vi "Retrieve Async Section configuration properties (interactions).vi"(8 "error in":errorcluster, 11 "section item ref in":T2 format="%.0x") -> (0 "error out":errorcluster, 1 "status channel configuration":map{string, map{string, i32}}(c390), 2 "data channel configuration":T1[](array[typedef]), 3 "section item ref out":T2 format="%.0x", 4 "Found":bool)   [LabVIEW 2019, in "HLA Custom Device System Explorer.lvlib"]
uses:
  HLA Custom Device System Explorer.lvlib
  <vilib>/NI VeriStand/Custom Device API/Custom Device Item Ref.ctl
  Shared/interaction_parameter_configuration.ctl
  Shared/Constants.vi
  <vilib>/NI VeriStand/Custom Device API/Get Item Property (String).vi
  <vilib>/NI VeriStand/Custom Device API/Custom Device API.lvlib
  Shared/HLA Custom Device Shared.lvlib
  <vilib>/NI VeriStand/Custom Device Tools/Custom Device Utility Library/Custom Device Utility Library.lvlib
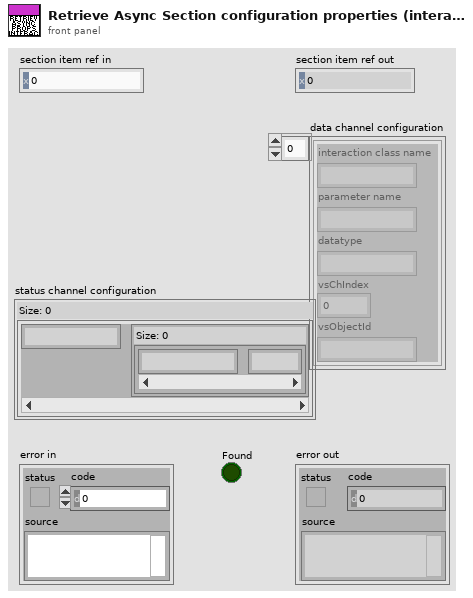
[diagram p1: front panel]
types:
  T1 = typedef "HLA Custom Device Shared.lvlib/interaction_parameter_configuration.ctl" = cluster{"interaction class name":string, "parameter name":string, "datatype":string, "vsChIndex":i32, "vsObjectId":string}
  T2 = typedef "Custom Device API.lvlib/Custom Device Item Ref.ctl" = u64
  T3 = typedef "Custom Device API.lvlib/Custom Device Item Info.ctl" = cluster{"Name":string, "Is Channel":bool, "GUID":string, "Is Waveform":bool}
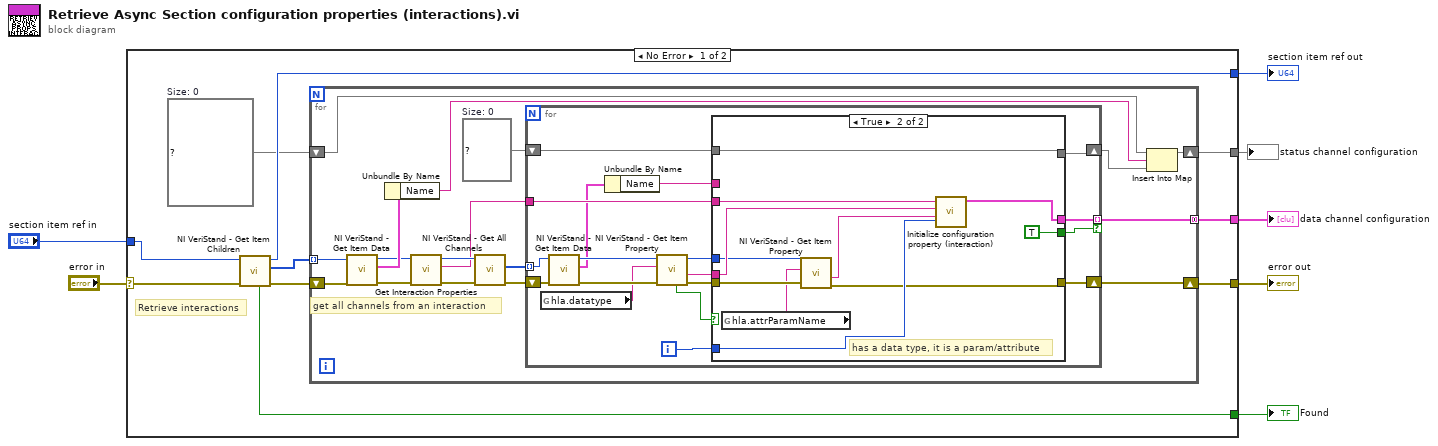
[diagram p0: block diagram]
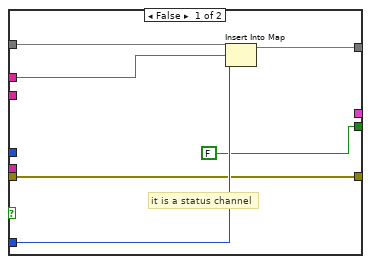
[diagram p2: hidden frame]
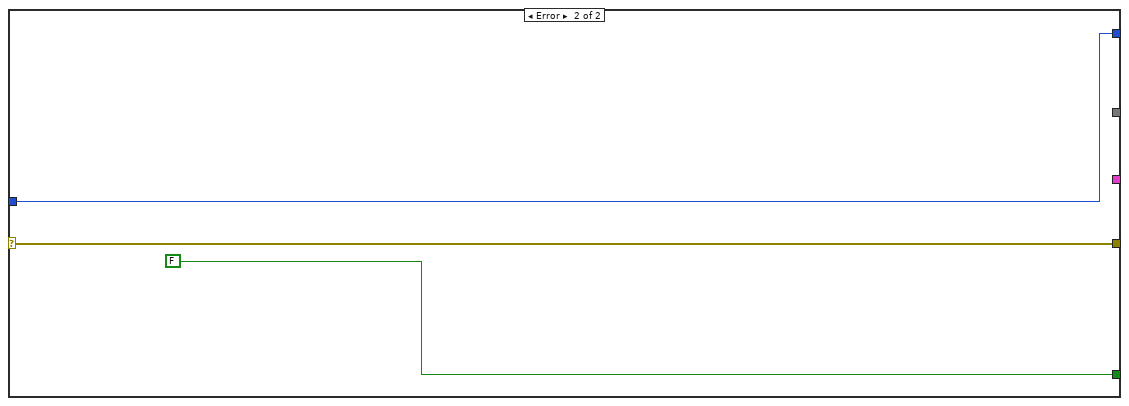
[diagram p3: hidden frame]
diagram:
  n1 = case shown="No Error" "error in" {
    selector: "error in" -> [w14 w71]
    tunnel: [w13 w71] -> w6
    tunnel: [w12 w72] -> w5
    tunnel: "section item ref in" -> [w15 w72]
    tunnel: [w10 FALSE ("Found")] -> w3
    tunnel: [w11 _] -> w2
    tunnel: [w8 _] -> w1
    frame No Error {
      w9 = map{string, map{string, i32}} {}  # Size: 0
      # "Retrieve interactions"
      n2 = call <vilib>:"NI VeriStand - Get Item Children.vi"("error in (no error)"=w14, "Item Ref in"=w15) -> ("error out"=w16:errorcluster, "Child Refs"=w17:T2[], "Item Ref out"=w12:T2, "Found"=w10:bool)  [unwired: 6 in]
      n3 = for {
        shift-right: [w30] -> w13
        shift-left: w16 -> [w33]
        tunnel: w17 -> [w32] mode=indexing
        tunnel: [w31] -> w11 mode=concatenating
        shift-right: [w24] -> w8
        shift-left: w9 -> [w25]
        w26 = map{string, i32} {}  # Size: 0
        # "get all channels from an interaction"
        n4 = call <vilib>:"NI VeriStand - Get Item Data.vi"("error in (no error)"=w33, "Item Ref in"=w32) -> ("error out"=w21:errorcluster, "Item Info"=w34:T3, "Item Ref out"=w29:T2)  [unwired: 6 in, 1 out]
        n5 = Unbundle By Name(w34) -> ("Name"=w18:string)
        n6 = call "Get Interaction Properties.vi"("error in (no error)"=w21, "Item Ref in"=w29) -> ("error out"=w20:errorcluster, "class name"=w19:string, "Item Ref out"=w22:T2)  [unwired: 7 in]
        n7 = call <vilib>:"NI VeriStand - Get All Channels.vi"("error in"=w20, "Section Ref in"=w22) -> ("error out"=w28:errorcluster, "Channel Refs"=w27:T2[])  [unwired: 6 in, 2 out]
        n8 = for {
          tunnel: w19 -> [w47]
          tunnel: w27 -> [w52] mode=indexing
          tunnel: [w46] -> w31 mode=indexing if=w39
          shift-right: [w37] -> w30
          shift-left: w28 -> [w51]
          shift-right: [w40] -> w23
          shift-left: w26 -> [w42]
          i -> [w41]
          n9 = global read "Constants.vi" "hla.datatype"() -> (w48:string)
          n10 = call <vilib>:"NI VeriStand - Get Item Data.vi"("error in (no error)"=w51, "Item Ref in"=w52) -> ("error out"=w49:errorcluster, "Item Info"=w44:T3, "Item Ref out"=w50:T2)  [unwired: 6 in, 1 out]
          n11 = Unbundle By Name(w44) -> ("Name"=w35:string)
          n12 = call-poly <vilib>:"NI VeriStand - Get Item Property.vi"("error in (no error)"=w49, "Property Name"=w48, "Item Ref in"=w50) -> ("error out"=w38:errorcluster, "Value"=w45:string, "Item Ref out"=w36:T2, "Found?"=w43:bool)  [unwired: 5 in]
          n13 = case shown="True" w43 {
            tunnel: w47 -> [_ w59]
            tunnel: [_ w69] -> w46
            tunnel: w45 -> [_ w68]
            tunnel: w42 -> [w58 w66]
            tunnel: w41 -> [w57 w65]
            tunnel: [w56 w66] -> w40
            tunnel: [FALSE TRUE] -> w39
            tunnel: w35 -> [w53 _]
            tunnel: w38 -> [w54 w64]
            tunnel: [w54 w63] -> w37
            tunnel: w36 -> [_ w62]
            frame False {
              # "it is a status channel"
              n14 = Insert Into Map(map in=w58, key=w53, value=w57) -> (map out=w56:map{string, i32})  [unwired: 2 out]
            }
            frame True {
              # "has a data type, it is a param/attribute"
              n15 = global read "Constants.vi" "hla.attrParamName"() -> (w61:string)
              n16 = call-poly <vilib>:"NI VeriStand - Get Item Property.vi"("error in (no error)"=w64, "Property Name"=w61, "Item Ref in"=w62) -> ("error out"=w63:errorcluster, "Value"=w60:string)  [unwired: 5 in, 2 out]
              n17 = call "Initialize configuration property (interaction).vi"("vsChIndex"=w65, "parameter name"=w60, "datatype"=w68, "interaction class name"=w59) -> ("attribute configuration"=w69:T1)  [unwired: 7 in]
            }
          }
        }
        n18 = Insert Into Map(map in=w25, key=w18, value=w23) -> (map out=w24:map{string, map{string, i32}})  [unwired: 2 out]
      }
    }
    frame Error {
    }
  }
  "error out" <- w6
  "section item ref out" <- w5
  "Found" <- w3
  "data channel configuration" <- w2
  "status channel configuration" <- w1
